vi "Ping 2013 NIVerified.vi"() -> ()   [LabVIEW 2013]
doc: "The program revolves around the usage of the Windows diagnostics tools available through the command \"arp -a\" and ping all of the IP.s from this command to see which ones are valid and place these into an array."
uses:
  StatesTypeDef.ctl
panel:
  in  "Gateway":string
  out "Output IP Addresses":string[](array[string])
  # "Overview: This code uses the .NET ping methods to ping all IP's collected from the Windows network diagnostics tool \nin the command prompt.\nRequirements: LabVIEW 2013 (or compatible), Windows Operating System\nInstructions:\n1. Input the Gateway , or left it empty.\n2. Run the VI."
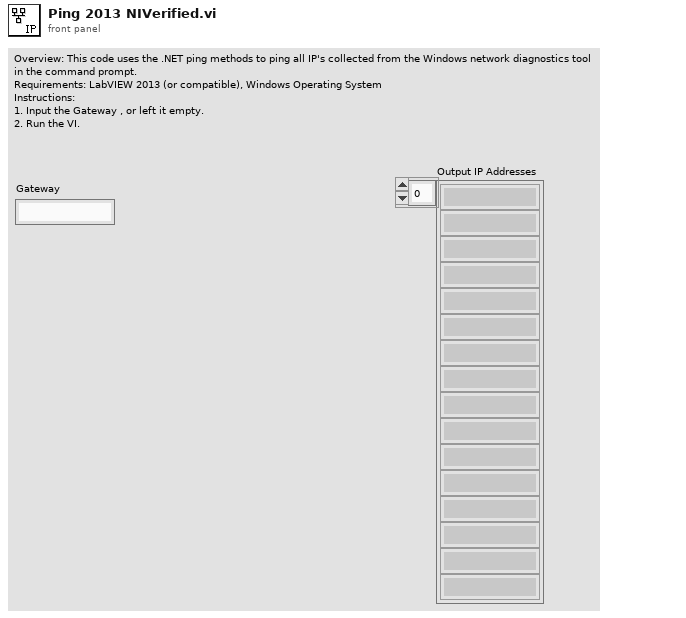
[diagram p1: front panel]
types:
  T1 = typedef "StatesTypeDef.ctl" = enum16{"Initialize", "TestGateway", "PingallPossibleIP's", "Exit"}
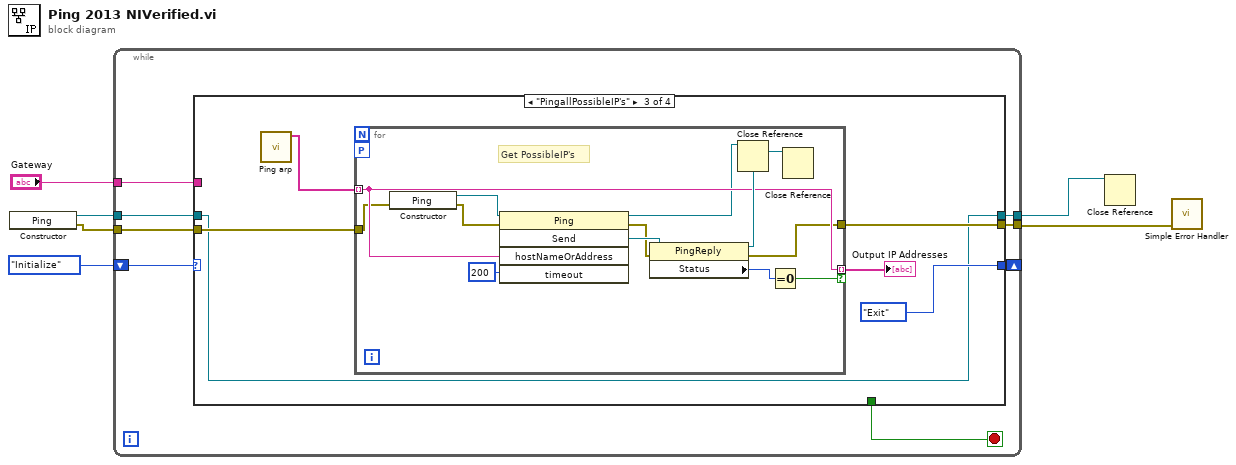
[diagram p0: block diagram]
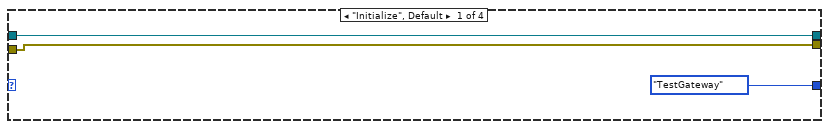
[diagram p2: hidden frame]
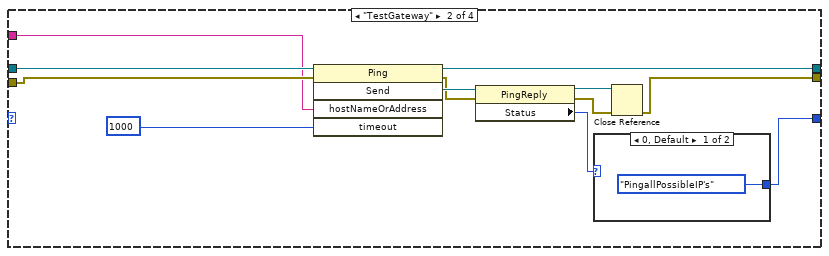
[diagram p3: hidden frame]
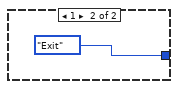
[diagram p4: hidden frame]
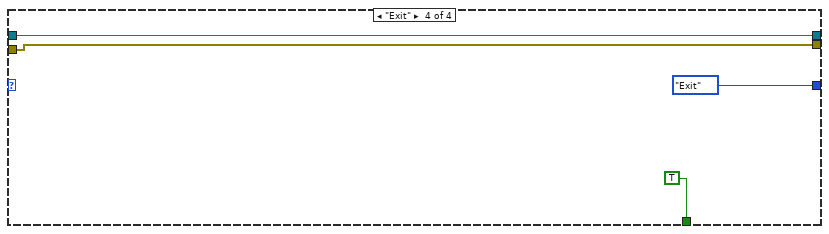
[diagram p5: hidden frame]
diagram:
  n1 = constructor class="Ping"() -> (reference out=w5:refnum<k24>, error out=w4:errorcluster)  [unwired: 3 in, 1 out]
  n2 = while {
    shift-right: [w14] -> _
    shift-left: StatesTypeDef."Initialize" ("Enum") -> [w13]
    tunnel: w5 -> [w12]
    tunnel: w4 -> [w11]
    tunnel: [w10] -> w3
    tunnel: [w9] -> w2
    tunnel: "Gateway" -> [w7]
    stop <- w8 stop-if-true
    n3 = case shown="\"PingallPossibleIP's\"" w13 {
      tunnel: [StatesTypeDef."TestGateway" ("Enum") w26 StatesTypeDef."Exit" ("Enum") StatesTypeDef."Exit" ("Enum")] -> w14
      tunnel: w7 -> [_ w18 _ _]
      tunnel: w12 -> [w17 w25 w33 w52]
      tunnel: [w17 w24 w33 w52] -> w9
      tunnel: w11 -> [w16 w23 w37 w51]
      tunnel: [w16 w20 w36 w51] -> w10
      tunnel: [_ _ _ TRUE] -> w8
      frame "Initialize", Default {
      }
      frame "TestGateway" {
        n4 = invoke class="Ping" method="Send"(reference=w25, error in=w23, "hostNameOrAddress"=w18, "timeout"=1000) -> (reference out=w24:refnum<k24>, error out=w22:errorcluster, "Send"=w29:refnum<k24>)  [unwired: 1 in, 2 out]
        n5 = property class="PingReply"(reference=w29, error in=w22) -> (reference out=w27:refnum<k24>, error out=w21:errorcluster, "Status"=w28:i32)
        n6 = case shown="0, Default" w28 {
          tunnel: [StatesTypeDef."PingallPossibleIP's" ("Enum") StatesTypeDef."Exit" ("Enum")] -> w26
          frame 0, Default {
          }
          frame 1 {
          }
        }
        n7 = Close Reference(reference=w27, error in (no error)=w21) -> (error out=w20:errorcluster)
      }
      frame "PingallPossibleIP's" {
        n8 = call "Ping arp.vi"() -> ("IP Addresses Output"=w32:string[])  [unwired: 11 in]
        n9 = for {
          tunnel: w37 -> [w41]
          tunnel: [w38] -> w36
          tunnel: w32 -> [w44] mode=indexing
          tunnel: [w44] -> w34 mode=indexing if=w47
          workers-P: _ -> [_]
          # "Get PossibleIP's"
          n10 = constructor class="Ping"(error in=w41) -> (reference out=w43:refnum<k24>, error out=w42:errorcluster)  [unwired: 2 in, 1 out]
          n11 = invoke class="Ping" method="Send"(reference=w43, error in=w42, "hostNameOrAddress"=w44, "timeout"=200) -> (reference out=w40:refnum<k24>, error out=w39:errorcluster, "Send"=w49:refnum<k24>)  [unwired: 1 in, 2 out]
          n12 = property class="PingReply"(reference=w49, error in=w39) -> (reference out=w45:refnum<k24>, error out=w38:errorcluster, "Status"=w48:i32)
          n13 = Close Reference(reference=w40) -> ()  [unwired: 1 in, 1 out]
          n14 = Equal To 0?(x=w48) -> (x = 0?=w47:bool)
          n15 = Close Reference(reference=w45) -> ()  [unwired: 1 in, 1 out]
        }
        "Output IP Addresses" <- w34
      }
      frame "Exit" {
      }
    }
  }
  n16 = Close Reference(reference=w2) -> ()  [unwired: 1 in, 1 out]
  n17 = call <vilib>:"Simple Error Handler.vi"("error in (no error)"=w3) -> ()  [unwired: 4 in, 5 out]
